vi "Configure Is Receive Filter.vi"(8 "error in (no error)":errorcluster, 10 "Show Receive?":bool, 11 "Debugger In":refnum<class "Debugger.lvclass">) -> (0 "error out":errorcluster, 3 "Debugger Out":refnum<class "Debugger.lvclass">)   [LabVIEW 2020, in "Debugger.lvclass"]
uses:
  Debugger.lvclass
  C:/Users/anton/Documents/GitHub/triarc-debugger/source/Process/Debug Process.lvclass
  Process/Debug Process.lvclass/Debug Process.ctl
  Debugger.lvclass/Debugger.ctl
  <vilib>/Utility/error.llb/Clear Errors.vi
  Filter by Is Receive/Filter by Is Receive.lvclass
  C:/Users/anton/Documents/GitHub/triarc-debugger/source/Filter/Filter.lvclass
  <vilib>/Utility/error.llb/Error Cluster From Error Code.vi
  Process/Debug Process.lvclass
  Debug Log/Debug Log.lvclass
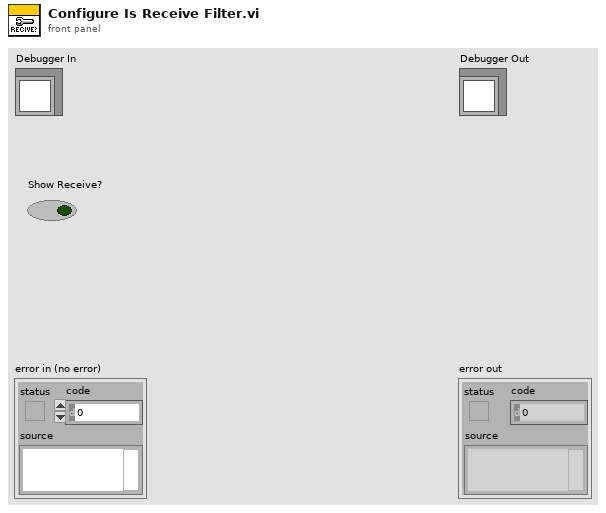
[diagram p1: front panel]
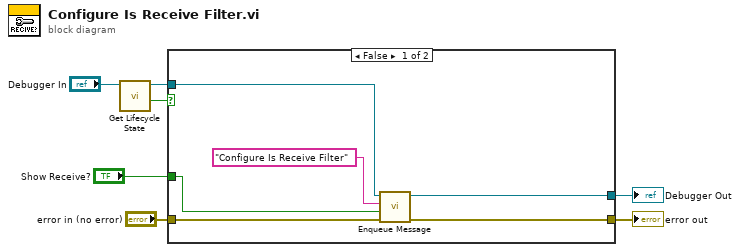
[diagram p0: block diagram]
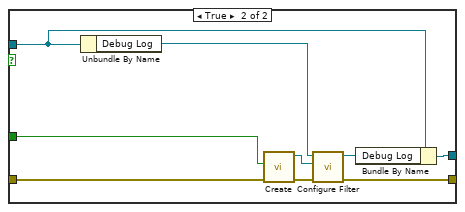
[diagram p2: hidden frame]
diagram:
  n1 = call "Get Lifecycle State.vi"("Process In"="Debugger In") -> ("In Process Loop?"=w2:bool, "Process Out"=w3:refnum<class "Debugger.lvclass">)  [unwired: 7 in, 2 out]
  n2 = case shown="False" w2 {
    tunnel: "error in (no error)" -> [w13 w20]
    tunnel: [w12 w19] -> w6
    tunnel: [w11 w21] -> w4
    tunnel: w3 -> [w9 w22]
    tunnel: "Show Receive?" -> [w8 w14]
    frame False {
      n3 = call "Enqueue Message.vi"("error in (no error)"=w13, "Message Data"=w8, "Message"="Configure Is Receive Filter", "Process In"=w9) -> ("error out"=w12:errorcluster, "Process Out"=w11:refnum<class "Debugger.lvclass">)  [unwired: 6 in]
    }
    frame True {
      n4 = Unbundle By Name(w22) -> ("Debug Log"=w18:refnum<class "Debug Log.lvclass">)
      n5 = call "Create.vi"("error in (no error)"=w20, "Show Receive?"=w14) -> ("error out"=w16:errorcluster, "Filter by Process out"=w17:refnum<class "Filter by Is Receive.lvclass">)  [unwired: 8 in]
      n6 = call "Configure Filter.vi"("error in (no error)"=w16, "Filter"=w17, "Debug Log In"=w18) -> ("error out"=w19:errorcluster, "Debug Log Out"=w15:refnum<class "Debug Log.lvclass">)  [unwired: 7 in]
      n7 = Bundle By Name(cluster=w22, "Debug Log"=w15) -> (w21:refnum<class "Debugger.lvclass">)
    }
  }
  "error out" <- w6
  "Debugger Out" <- w4
